vi "mqttCmdMessageIDWrite.vi"(0 "mqttBrokerCommand in":refnum<class "mqttCmd.lvclass">, 5 "messageID":u16, 11 "error in (no error)":errorcluster) -> (4 "mqttBrokerCommand out":refnum<class "mqttCmd.lvclass">, 15 "error out":errorcluster)   [LabVIEW 2020, in "mqttCmd.lvclass"]
uses:
  mqttCmd.lvclass
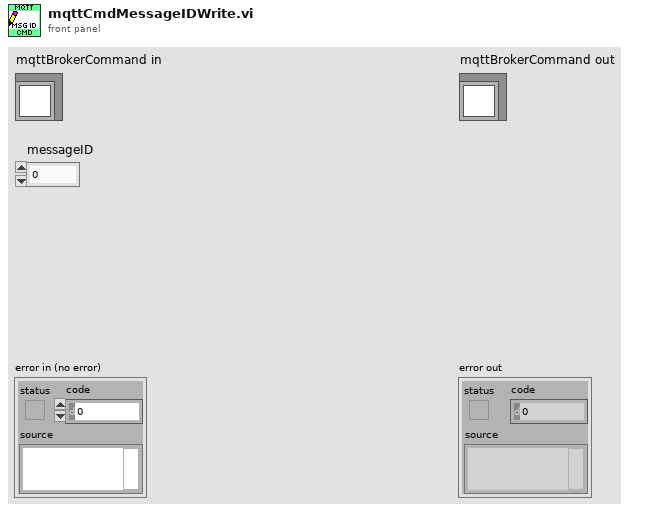
[diagram p1: front panel]
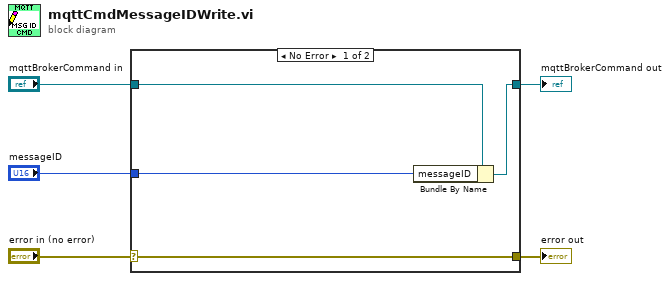
[diagram p0: block diagram]
diagram:
  n1 = case shown="No Error" "error in (no error)" {
    selector: "error in (no error)" -> [w9 w10]
    tunnel: [w9 w10] -> w4
    tunnel: [w7 w11] -> w2
    tunnel: "mqttBrokerCommand in" -> [w8 w11]
    tunnel: "messageID" -> [w6 _]
    frame No Error {
      n2 = Bundle By Name(cluster=w8, "messageID"=w6) -> (w7:refnum<class "mqttCmd.lvclass">)
    }
    frame Error {
    }
  }
  "error out" <- w4
  "mqttBrokerCommand out" <- w2
